vi "SpolRVP8Pwr.vi"(6 "SpecifyTypeOfDataAcq":string="_", 7 "DataSource":bool, 8 "error in (no error)":errorcluster, 9 "startGate":i32=200 min=1025 step=1, 10 "nGates":i32=500 min=1025 step=1, 11 "nSamples":i32=1000) -> (0 "Comm error":errorcluster, 1 "XML error":errorcluster, 2 "String_of_RVP8_Powers":string, 3 "RVP8_power":T1 {"time" format="%<%H:%M:%S\n%Y/%m/%d>T"})   [LabVIEW 2012]
doc: "Reads the power from the N1911A power meter."
uses:
  Rvp8PowerData.ctl
panel:
  out "XML Response":string="fetch?"
  out "XML commands":string="<TsGrabberCommands>\n  <nSamples>1000</nSamples>\n  <startGate>50</startGate>\n  <nGates>500</nGates>\n  <fastAlternating>true</fastAlternating>\n  <labviewRequest>true</labviewRequest>\n</TsGrabberCommands>\n"
  # "Changed StartGate and nGates to I32 and corrected wiring to each of these (fp:17Aug07).  The defaults must be 1000/500/50 for the calibration programs to work correctly!"
  # "Select ngates and startgate to avoid standard test pulse and Rx switching transient"
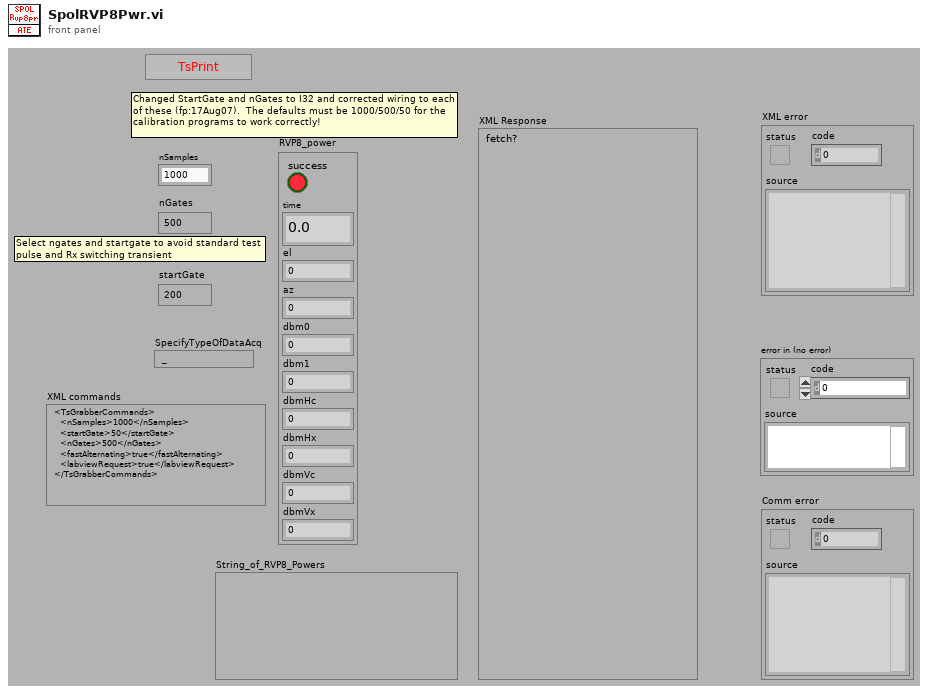
[diagram p1: front panel]
types:
  T1 = typedef "Rvp8PowerData.ctl" = cluster{"success":bool, "time":dbl, "el":dbl, "az":dbl, "dbm0":dbl, "dbm1":dbl, "dbmHc":dbl, "dbmHx":dbl, "dbmVc":dbl, "dbmVx":dbl}
  T2 = enum16{"N1911A", "Siggen", "34980a", "E4418B", "Rvp8"}
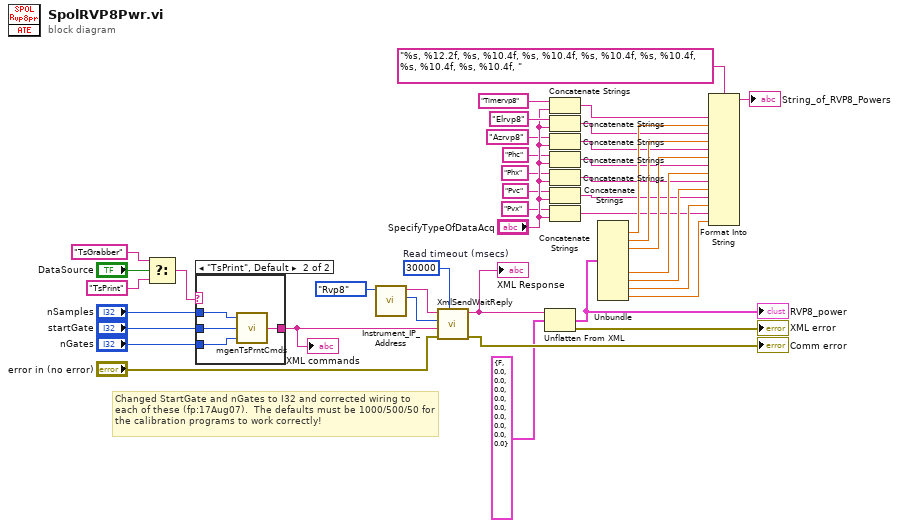
[diagram p0: block diagram]
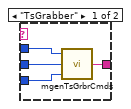
[diagram p2: hidden frame]
diagram:
  w39 = 30000  # Read timeout (msecs)
  # "Changed StartGate and nGates to I32 and corrected wiring to each of these (fp:17Aug07).  The defaults must be 1000/500/50 for the calibration programs to work correctly!"
  n1 = Select(t="TsGrabber", s="DataSource", f="TsPrint") -> (s? t:f=w3:string)
  n2 = case shown="\"TsPrint\", Default" w3 {
    tunnel: [w46 w50] -> w35
    tunnel: "nSamples" -> [w44 w49]
    tunnel: "startGate" -> [w45 w48]
    tunnel: "nGates" -> [w43 w47]
    frame "TsGrabber" {
      n3 = call "mgenTsGrbrCmds.vi"("nGates"=w43, "startGate"=w45, "nSamples"=w44) -> ("TsGrabberCommand"=w46:string)
    }
    frame "TsPrint", Default {
      n4 = call "mgenTsPrntCmds.vi"("nGates"=w47, "startGate"=w48, "nSamples"=w49) -> ("TsPrintCommand"=w50:string)
    }
  }
  "XML commands" <- w35
  n5 = call "Instrument_IP_Address.vi"("Instrument"=T2."Rvp8") -> ("Port"=w41:u16, "IP Address"=w40:string)  [unwired: 9 in]
  n6 = call "XmlSendWaitReply.vi"("Read timeout msecs"=w39, "error in (no error)"="error in (no error)", "Command"=w35, "TCP port"=w41, "IP Address"=w40) -> ("Error out"=→"Comm error":errorcluster, "Reply"=w6:string)  [unwired: 4 in]
  "XML Response" <- w6
  n7 = Unflatten From XML(xml string=w6, type=T1 {"success"=FALSE, "time"=0.0, "el"=0.0, "az"=0.0, "dbm0"=0.0, "dbm1"=0.0, "dbmHc"=0.0, "dbmHx"=0.0, "dbmVc"=0.0, "dbmVx"=0.0} ("RVP8_power 2")) -> (value=w30:T1, error out=→"XML error":errorcluster)  [unwired: 1 in]
  "RVP8_power" <- w30
  n8 = Concatenate Strings("Timervp8", "SpecifyTypeOfDataAcq") -> (w16:string)
  n9 = Concatenate Strings("Elrvp8", "SpecifyTypeOfDataAcq") -> (w15:string)
  n10 = Concatenate Strings("Azrvp8", "SpecifyTypeOfDataAcq") -> (w14:string)
  n11 = Concatenate Strings("Phc", "SpecifyTypeOfDataAcq") -> (w12:string)
  n12 = Concatenate Strings("Phx", "SpecifyTypeOfDataAcq") -> (w11:string)
  n13 = Concatenate Strings("Pvc", "SpecifyTypeOfDataAcq") -> (w10:string)
  n14 = Concatenate Strings("Pvx", "SpecifyTypeOfDataAcq") -> (w9:string)
  n15 = Unbundle(w30) -> ("time"=w29:dbl, "el"=w28:dbl, "az"=w13:dbl, "dbmHc"=w27:dbl, "dbmHx"=w26:dbl, "dbmVc"=w25:dbl, "dbmVx"=w24:dbl)  [unwired: 3 out]
  n16 = Format Into String(format string="%s, %12.2f, %s, %10.4f, %s, %10.4f, %s, %10.4f, %s, %10.4f, %s, %10.4f, %s, %10.4f, ", w16, w29, w15, w28, w14, w13, w12, w27, w11, w26, w10, w25, w9, w24) -> (resulting string=→"String_of_RVP8_Powers":string)  [unwired: 2 in, 1 out]
